vi "Copy Value.vi"(8 "error in (no error)":errorcluster, 10 "From":refnum<class "Type.lvclass">, 11 "Type in":refnum<class "Type.lvclass">) -> (0 "error out":errorcluster, 3 "Type out":refnum<class "Type.lvclass">)   [LabVIEW 2020, in "Conditum.lvlib" / "Columns.lvlib" / "Type.lvclass"]
uses:
  Type.lvclass
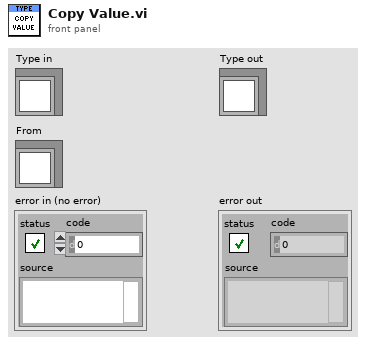
[diagram p1: front panel]
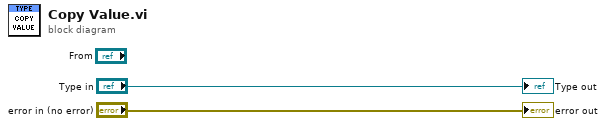
[diagram p0: block diagram]
diagram:
  "error out" <- "error in (no error)"
  "Type out" <- "Type in"
